vi "NI VeriStand - Synchronize to Host.vi"(1 "Clock Ticked":bool, 2 "Generate IRQ":bool) -> (0 "Is Late?":u64)   [LabVIEW 2010, in "NI_VS FPGA Clock Support.lvlib"]
uses:
  <userlib>/_NI VeriStand FPGA Support/NI VeriStand FPGA Clock Support/NI_VS FPGA Clock Support.lvlib
  <userlib>/_NI VeriStand FPGA Support/NI VeriStand FPGA Clock Support/NI VeriStand - Timing Engine Globals.vi
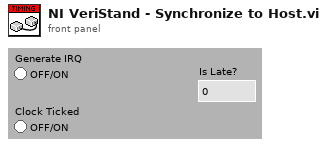
[diagram p1: front panel]
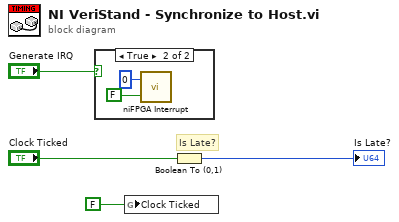
[diagram p0: block diagram]
diagram:
  # "Is Late?"
  n1 = case shown="True" "Generate IRQ" {
    frame False {
    }
    frame True {
      n2 = call <vilib>:"niFPGA Interrupt.vi"("Wait Until Cleared"=FALSE, "IRQ Number"=u8 0) -> ()  [unwired: 1 in]
    }
  }
  n3 = global write "NI VeriStand - Timing Engine Globals.vi" "Clock Ticked"(FALSE ("Clock Ticked")) -> ()
  n4 = Boolean To (0,1)(Boolean="Clock Ticked") -> (0, 1=→"Is Late?":i16)
